vi "encoding_matlab.vi"(0 "d":dbl, 5 "y0":dbl, 7 "y1":dbl) -> (4 "modes":dbl[](array[numeric]), 6 "coeffs":dbl[](array[numeric]), 8 "phase":dbl[](array[numeric]))   [LabVIEW 2015]
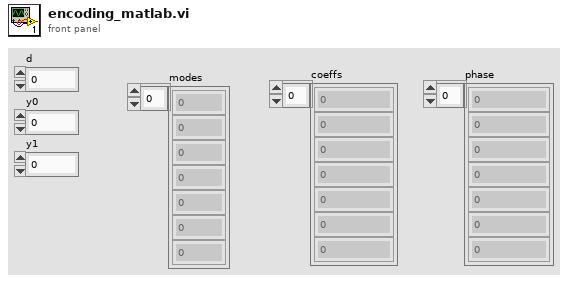
[diagram p1: front panel]
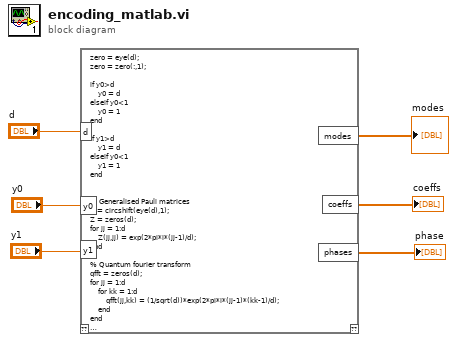
[diagram p0: block diagram]
diagram:
  n1 = script code="zero = eye(d);\nzero = zero(:,1);\n\nif y0>d \n    y0 = d\nelseif y0<1\n    y0 = 1\nend\n\nif y1>d \n    y1 = d\nelseif y0<1\n    y1 = 1\nend\n\n\n% Generalised Pauli matrices\nX = circshift(eye(d),1);\nZ = zeros(d);\nfor jj = 1:d\n    Z(jj,jj) = exp(2*pi*i*(jj-1)/d);\nend\n\n% Quantum fourier transform\nqfft = zeros(d);\nfor jj = 1:d\n    for kk = 1:d\n        qfft(jj,kk) = (1/sqrt(d))*exp(2*pi*i*(jj-1)*(kk-1)/d);\n    end\nend\n\nencode = (1/sqrt(2+(2/sqrt(d))))*(X^(y0-1))*(Z^(y1-1))*(zero+qfft*zero);\nmodes = [round(linspace(floor(d/2),-floor(d/2),d))]\ncoeffs = [abs(encode)]'\nphases = [angle(encode)]'"("d"="d", "y0"="y0", "y1"="y1") -> ("modes"=→"modes":dbl[], "coeffs"=→"coeffs":dbl[], "phases"=→"phase":dbl[])  [unwired: 1 in, 1 out]
